vi "Channel configuration UI.vi"(11 "config file":path) -> (0 "updated?":bool, 3 "Current config file:":path)   [LabVIEW 2018]
uses:
  ICL-LabVIEW_General/data channels/parent class/Supporting functions/channel display control.ctl
  ICL-LabVIEW_General/data channels/parent class/channel type.ctl
  ICL-LabVIEW_General/data channels/parent class/Supporting functions/scaling types.ctl
  ICL-LabVIEW_General/data channels/parent class/dataSource.ctl
  channel config UI states.ctl
  RT/Type Defs/channelScalingTypes.ctl
  ICL-LabVIEW_General/data channels/parent class/Data Channel.lvclass
  ICL-LabVIEW_General/data channels/data channels.lvlib
panel:
  in  "Filter:":T1(ring)
  in  "channelSettings":T2[](array[typedef])
  in  "reset":bool
  in  "load":bool
  in  "save as":bool
  in  "save":bool
  in  "cancel":bool
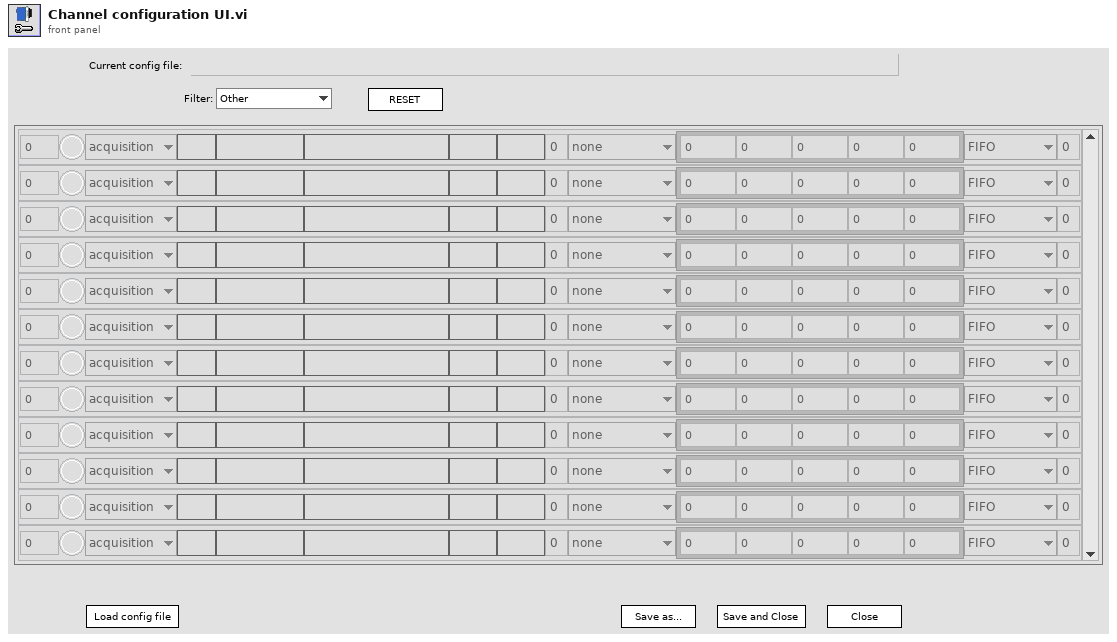
[diagram p1: front panel]
types:
  T1 = enum16{"Other", "Module 1", "Module 2", "Module 3", "Module 4", "Module 5", "Module 6", "Module 7", "Module 8", "Scanivalve", "All"}
  T2 = typedef "data channels.lvlib/channel display control.ctl" = cluster{"index":u16, "active":bool, "channelType":T3, "module":string, "terminal":string, "channelName":string, "unscaledUnits":string, "scaledUnits":string, "precision":u8, "scalingMethod":T4, "scalingParameters":dbl[], "liveOffset":dbl, "dataSource":T5, "FIFOIndex":u8}
  T3 = typedef "data channels.lvlib/Data Channel.lvclass/channel type.ctl" = enum16{"acquisition", "output", "other"}
  T4 = typedef "data channels.lvlib/scaling types.ctl" = enum16{"none", "linear", "thermocouple", "polynomial", "encoder", "RTD", "V-Cone", "pressureRatio"}
  T5 = typedef "data channels.lvlib/Data Channel.lvclass/dataSource.ctl" = enum16{"Not available", "FIFO", "Scanivalve", "Remote", "Calculated"}
  T6 = typedef "channel config UI states.ctl" = enum16{"wait", "load", "init", "filter", "save", "save as", "close"}
  T7 = typedef "channelScalingTypes.ctl" = enum16{"calculation", "measurement", "scanivalve", "output", "digital"}
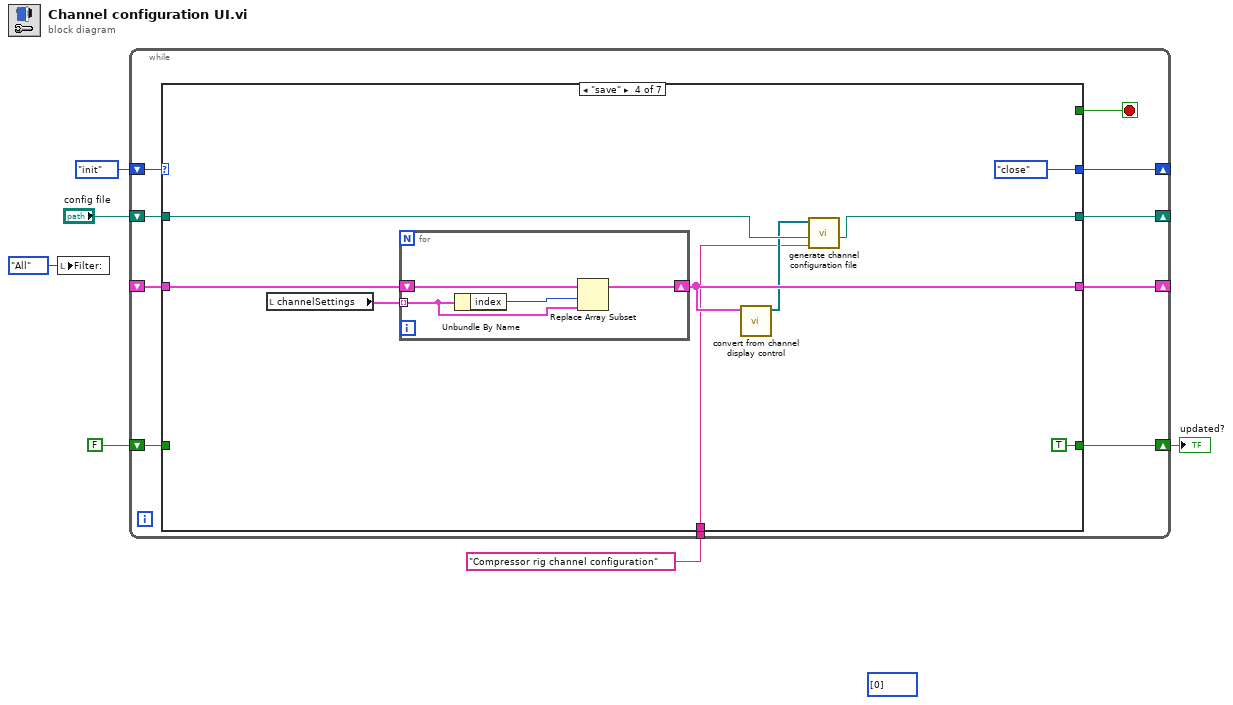
[diagram p0: block diagram]
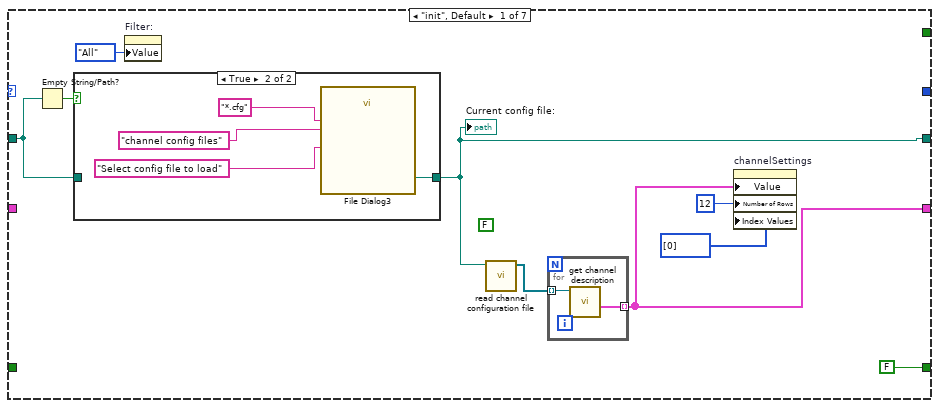
[diagram p2: hidden frame]
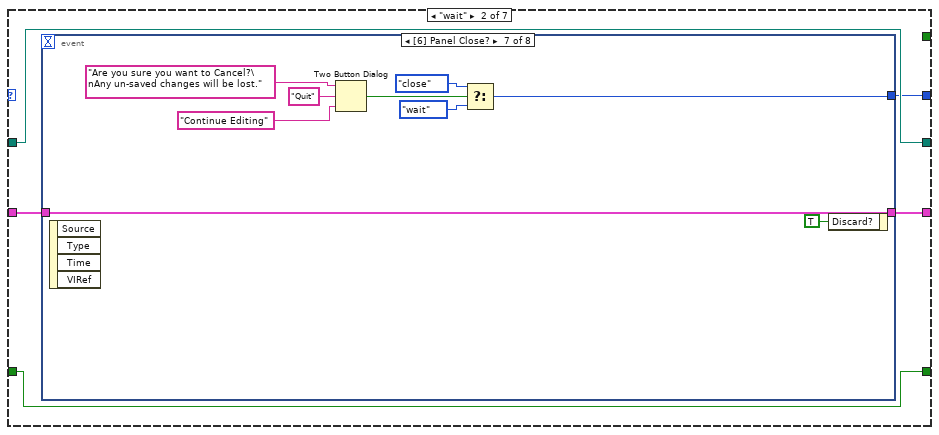
[diagram p4: hidden frame]
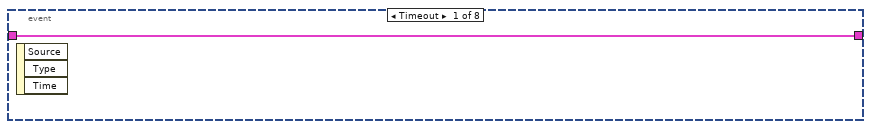
[diagram p5: hidden frame]
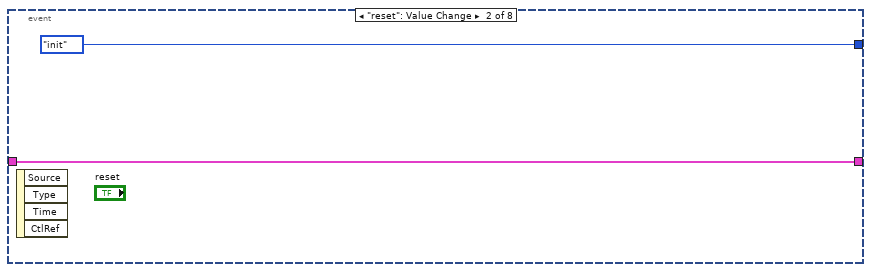
[diagram p6: hidden frame]
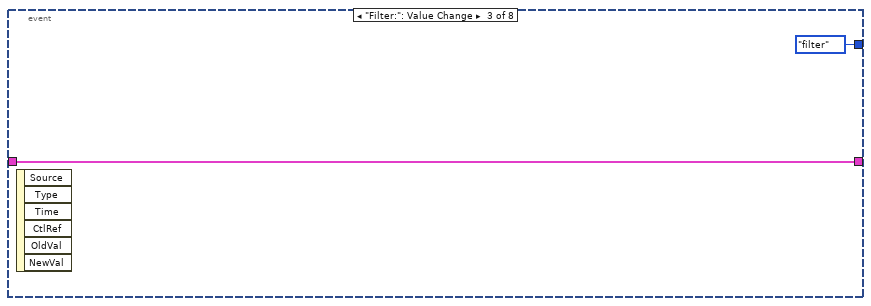
[diagram p7: hidden frame]
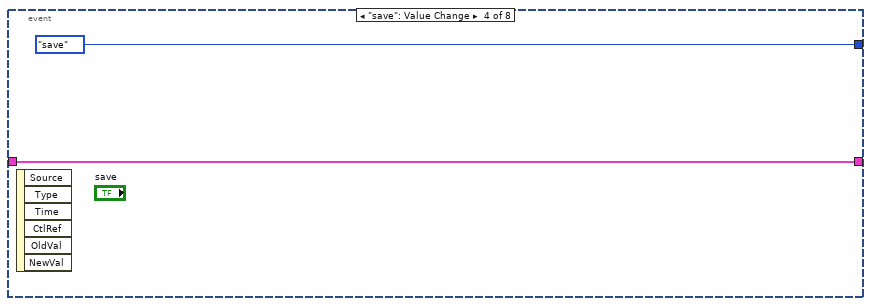
[diagram p8: hidden frame]
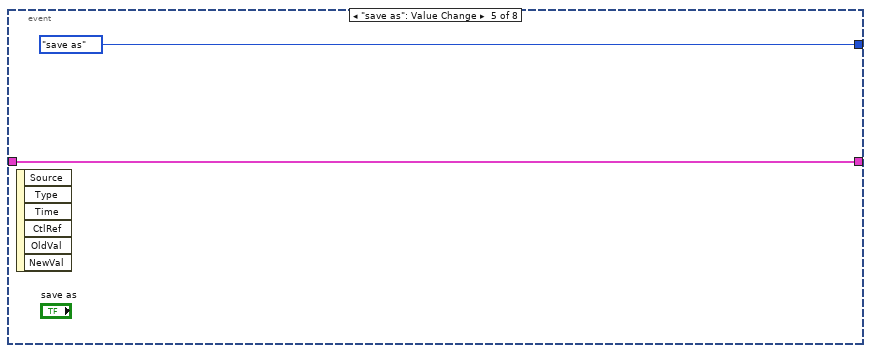
[diagram p9: hidden frame]
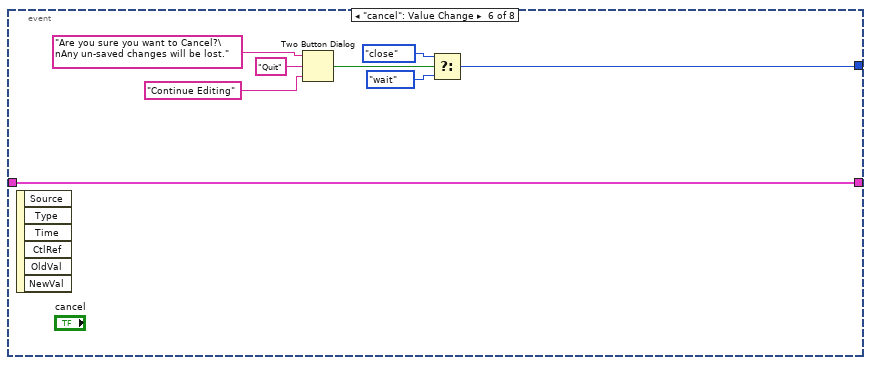
[diagram p10: hidden frame]
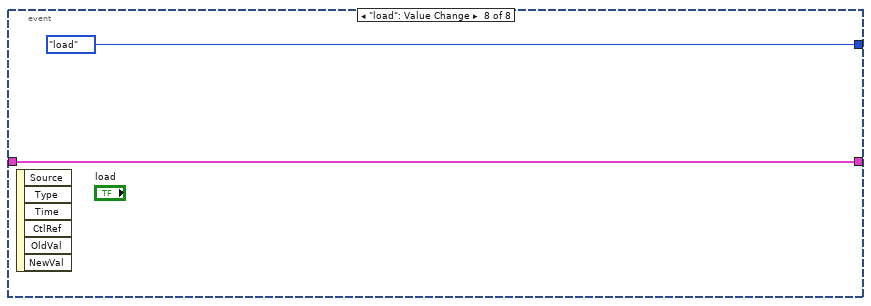
[diagram p11: hidden frame]
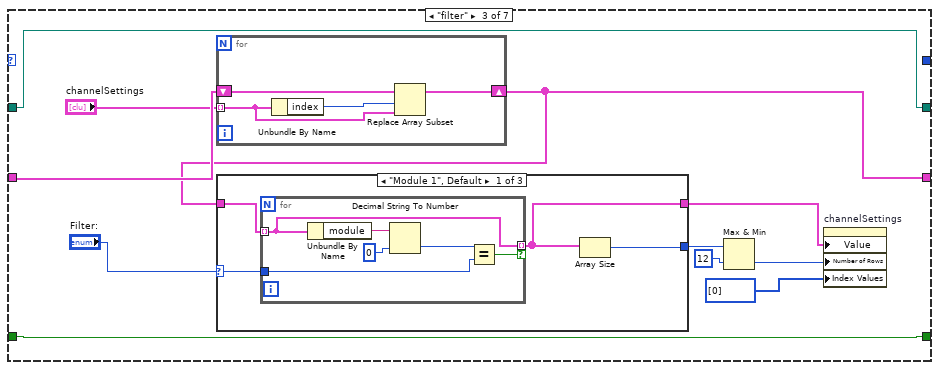
[diagram p12: hidden frame]
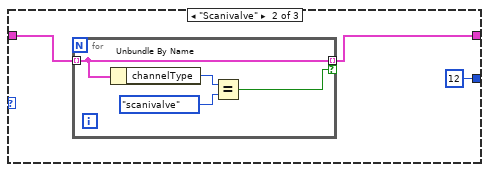
[diagram p13: hidden frame]
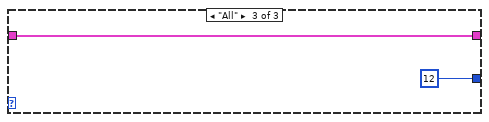
[diagram p14: hidden frame]
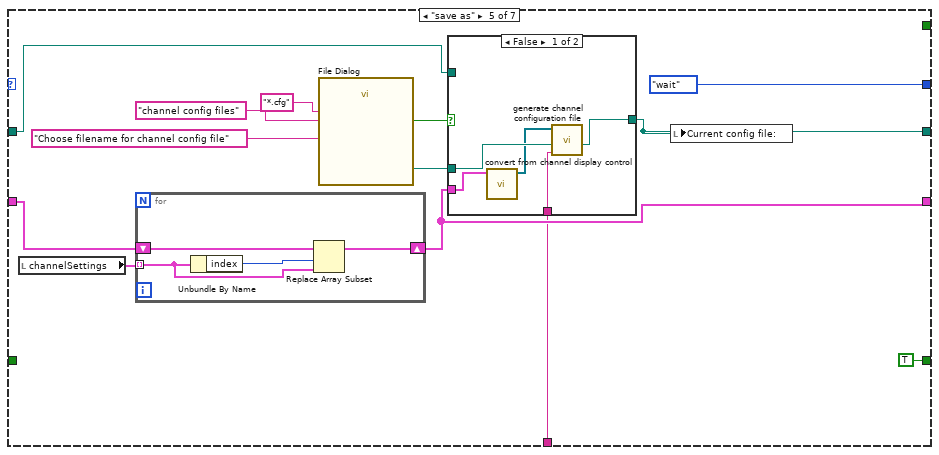
[diagram p15: hidden frame]
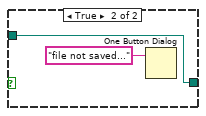
[diagram p16: hidden frame]
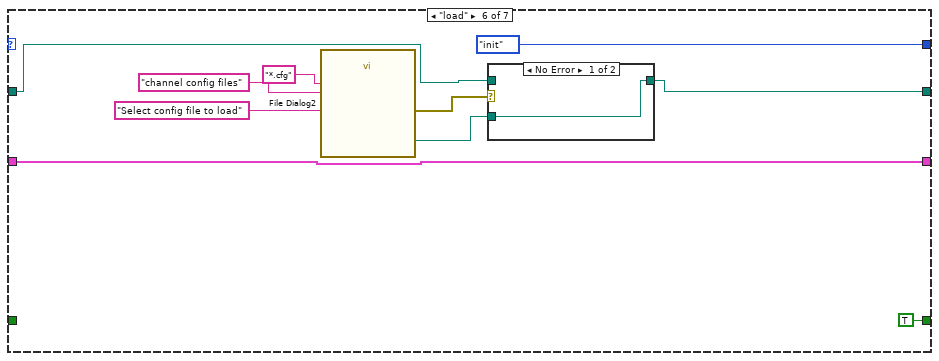
[diagram p17: hidden frame]
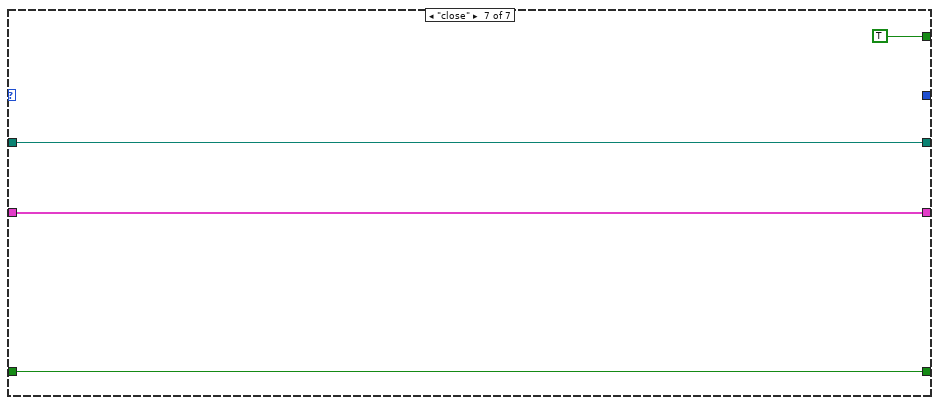
[diagram p19: hidden frame]
diagram:
  (unwired) u32[] [0] ("Index Values")
  n1 = local write "Filter:"(T1."All" ("Filter:")) -> ()
  n2 = while {
    shift-right: [w15] -> _
    shift-left: _ -> [w16]
    shift-right: [w11] -> _
    shift-left: "config file" -> [w13]
    shift-right: [w10] -> _
    shift-left: channel_config_UI_states."init" -> [w12]
    shift-right: [w8] -> w2
    shift-left: FALSE -> [w9]
    tunnel: "Compressor rig channel configuration" ("custom config file title") -> [w7]
    stop <- w14 stop-if-true
    n3 = case shown="\"save\"" w12 {
      tunnel: w16 -> [_ w37 w74 w107 w116 w142 w151]
      tunnel: [w17 w36 w66 w102 w115 w142 w151] -> w15
      tunnel: [_ _ _ _ _ _ TRUE ("cancel")] -> w14
      tunnel: w13 -> [w22 w35 w68 w104 w119 w139 w150]
      tunnel: [w19 w35 w68 w103 w118 w140 w150] -> w11
      tunnel: [_ w34 _ channel_config_UI_states."close" channel_config_UI_states."wait" channel_config_UI_states."init" _] -> w10
      tunnel: w9 -> [_ w33 w67 _ _ _ w149]
      tunnel: [FALSE w33 w67 TRUE TRUE TRUE w149] -> w8
      tunnel: w7 -> [_ _ _ w100 w113 _ _]
      frame "init", Default {
        (unwired) FALSE ("include lab ambient? (T)")
        n4 = Empty String/Path?(string/path=w22) -> (empty?=w23:bool)
        n5 = case shown="True" w23 {
          tunnel: w22 -> [w28 _]
          tunnel: [w28 w32] -> w19
          frame False {
          }
          frame True {
            n6 = call "File Dialog3"("prompt"="Select config file to load", "pattern (all files)"="*.cfg" ("pattern label"), "pattern label"="channel config files") -> ("selected path"=w32:path)  [unwired: 9 in, 3 out]
          }
        }
        "Current config file:" <- w19
        n7 = property on="Filter:" class="Enum (strict)"("Value"=T1."All" ("Filter:")) -> ()  [unwired: 2 in, 2 out]
        n8 = call "read channel configuration file.vi"("config file"=w19) -> ("channelsArray"=w18:refnum<class "Data Channel.lvclass">[])  [unwired: 8 in, 2 out]
        n9 = for {
          tunnel: w18 -> [w27] mode=indexing
          tunnel: [w26] -> w17 mode=indexing
          n10 = call-dynamic "get channel description.vi"("Data Channel in"=w27) -> ("channelScaling"=w26:T2)  [unwired: 7 in, 3 out]
        }
        n11 = property on="channelSettings" class="Arr (strict)"("Value"=w17, "Number of Rows"=u32 12, "Index Values"=u32[] [0]) -> ()  [unwired: 2 in, 2 out]
      }
      frame "wait" {
        n12 = event shown="[6] Panel Close?" {
          selector: _ -> [_ _ _ _ _ _ _ _]
          dyn-events: _ -> [_ _ _ _ _ _ _ _]
          timeout: _ -> [_ _ _ _ _ _ _ _]
          tunnel: w37 -> [w38 w39 w42 w44 w46 w54 w63 w65]
          tunnel: [w38 w39 w42 w44 w46 w54 w63 w65] -> w36
          tunnel: [_ channel_config_UI_states."init" channel_config_UI_states."filter" channel_config_UI_states."save" channel_config_UI_states."save as" w50 w59 channel_config_UI_states."load"] -> w34
          event Timeout {
            n13 = event-data() -> ()  [unwired: 1 in, 3 out]
          }
          event "reset": Value Change {
            n14 = event-data() -> ()  [unwired: 1 in, 4 out]
          }
          event "Filter:": Value Change {
            n15 = event-data() -> ()  [unwired: 1 in, 6 out]
          }
          event "save": Value Change {
            n16 = event-data() -> ()  [unwired: 1 in, 6 out]
          }
          event "save as": Value Change {
            n17 = event-data() -> ()  [unwired: 1 in, 6 out]
          }
          event "cancel": Value Change {
            n18 = event-data() -> ()  [unwired: 1 in, 6 out]
            n19 = Two Button Dialog(message="Are you sure you want to Cancel?\nAny un-saved changes will be lost.", 1:"Continue Editing" ("F button name (\"Cancel\")"), 2:"Quit" ("T button name (\"OK\")")) -> (T button?=w53:bool)
            n20 = Select(t=channel_config_UI_states."close", s=w53, f=channel_config_UI_states."wait") -> (s? t:f=w50:T6)
          }
          event Panel Close? {
            n21 = event-data() -> ()  [unwired: 1 in, 4 out]
            n22 = Two Button Dialog(message="Are you sure you want to Cancel?\nAny un-saved changes will be lost.", 1:"Continue Editing" ("F button name (\"Cancel\")"), 2:"Quit" ("T button name (\"OK\")")) -> (T button?=w62:bool)
            n23 = Select(t=channel_config_UI_states."close", s=w62, f=channel_config_UI_states."wait") -> (s? t:f=w59:T6)
            n24 = event-data("Discard?"=TRUE) -> ()  [unwired: 1 in, 1 out]
          }
          event "load": Value Change {
            n25 = event-data() -> ()  [unwired: 1 in, 6 out]
          }
        }
      }
      frame "filter" {
        n26 = for {
          tunnel: "channelSettings" -> [w78] mode=indexing
          shift-right: [w77] -> w66
          shift-left: w74 -> [w80]
          n27 = Unbundle By Name(w78) -> ("index"=w79:u16)
          n28 = Replace Array Subset(array=w80, new element=w78, index=w79) -> (w77:T2[])
        }
        n29 = case shown="\"Module 1\", Default" "Filter:" {
          selector: "Filter:" -> [w82 _ _]
          tunnel: w66 -> [w84 w93 w99]
          tunnel: [w83 w92 w99] -> w72
          tunnel: [w81 12 12 ("Number of Rows")] -> w75
          frame "Module 1", Default {
            n30 = for {
              tunnel: w84 -> [w90] mode=indexing
              tunnel: w82 -> [w86]
              tunnel: [w90] -> w83 mode=indexing if=w89
              n31 = Unbundle By Name(w90) -> ("module"=w88:string)
              n32 = Decimal String To Number(string=w88, default (0L)=u16 0) -> (number=w87:u16)  [unwired: 1 in, 1 out]
              n33 = Equal?(x=w87, y=w86) -> (x = y?=w89:bool)
            }
            n34 = Array Size(array=w83) -> (size(s)=w81:i32)
          }
          frame "Scanivalve" {
            n35 = for {
              tunnel: w93 -> [w95] mode=indexing
              tunnel: [w95] -> w92 mode=indexing if=w94
              n36 = Unbundle By Name(w95) -> ("channelType"=w97:T3)
              n37 = Equal?(x=w97, y=channelScalingTypes."scanivalve" ("channelType")) -> (x = y?=w94:bool)
            }
          }
          frame "All" {
          }
        }
        n38 = Max & Min(x=w75, y=12 ("Number of Rows")) -> (min(x,y)=w71:i32)  [unwired: 1 out]
        n39 = property on="channelSettings" class="Arr (strict)"("Value"=w72, "Number of Rows"=w71, "Index Values"=u32[] [0]) -> ()  [unwired: 2 in, 2 out]
      }
      frame "save" {
        n40 = local read "channelSettings"() -> (w106:T2[])
        n41 = for {
          tunnel: w106 -> [w110] mode=indexing
          shift-right: [w109] -> w102
          shift-left: w107 -> [w112]
          n42 = Unbundle By Name(w110) -> ("index"=w111:u16)
          n43 = Replace Array Subset(array=w112, new element=w110, index=w111) -> (w109:T2[])
        }
        n44 = call "convert from channel display control.vi"("channelDisplayControls"=w102) -> ("channels"=w101:refnum<class "Data Channel.lvclass">[])  [unwired: 10 in]
        n45 = call "generate channel configuration file.vi"("custom config file title"=w100, "config file"=w104, "channels"=w101) -> ("path"=w103:path)  [unwired: 8 in]
      }
      frame "save as" {
        n46 = local read "channelSettings"() -> (w117:T2[])
        n47 = for {
          tunnel: w117 -> [w127] mode=indexing
          shift-right: [w126] -> w115
          shift-left: w116 -> [w129]
          n48 = Unbundle By Name(w127) -> ("index"=w128:u16)
          n49 = Replace Array Subset(array=w129, new element=w127, index=w128) -> (w126:T2[])
        }
        n50 = call "File Dialog"("prompt"="Choose filename for channel config file", "pattern (all files)"="*.cfg" ("pattern label"), "pattern label"="channel config files") -> ("selected path"=w122:path, "cancelled"=w120:bool)  [unwired: 9 in, 2 out]
        n51 = case shown="False" w120 {
          tunnel: w122 -> [w133 _]
          tunnel: [w132 w136] -> w118
          tunnel: w115 -> [w134 _]
          tunnel: w119 -> [_ w136]
          tunnel: w113 -> [w130 _]
          frame False {
            n52 = call "convert from channel display control.vi"("channelDisplayControls"=w134) -> ("channels"=w131:refnum<class "Data Channel.lvclass">[])  [unwired: 10 in]
            n53 = call "generate channel configuration file.vi"("custom config file title"=w130, "config file"=w133, "channels"=w131) -> ("path"=w132:path)  [unwired: 8 in]
          }
          frame True {
            n54 = One Button Dialog(message="file not saved...") -> ()  [unwired: 1 in, 1 out]
          }
        }
        n55 = local write "Current config file:"(w118) -> ()
      }
      frame "load" {
        n56 = call "File Dialog2"("prompt"="Select config file to load", "pattern (all files)"="*.cfg" ("pattern label"), "pattern label"="channel config files") -> ("selected path"=w138:path, "error out"=w141:errorcluster)  [unwired: 9 in, 2 out]
        n57 = case shown="No Error" w141 {
          tunnel: [w147 w148] -> w140
          tunnel: w139 -> [_ w148]
          tunnel: w138 -> [w147 _]
          frame No Error {
          }
          frame Error {
          }
        }
      }
      frame "close" {
      }
    }
  }
  "updated?" <- w2
